vi "UsuarioContrasena.vi"() -> ()   [LabVIEW 2020]
panel:
  in  "stop":bool
  in  "Table Control":string[][](table)
  in  "Contraseña":string
  in  "Nombre":string
  out "Confirmado":bool
  out "Nombre confirmado":string
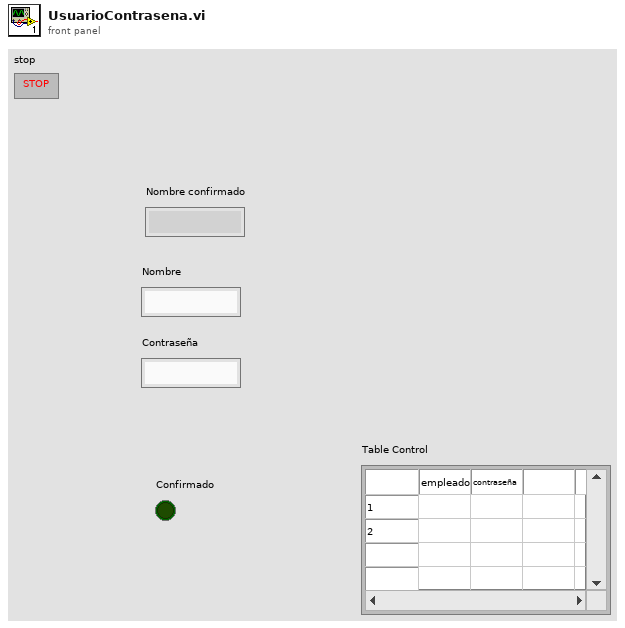
[diagram p1: front panel]
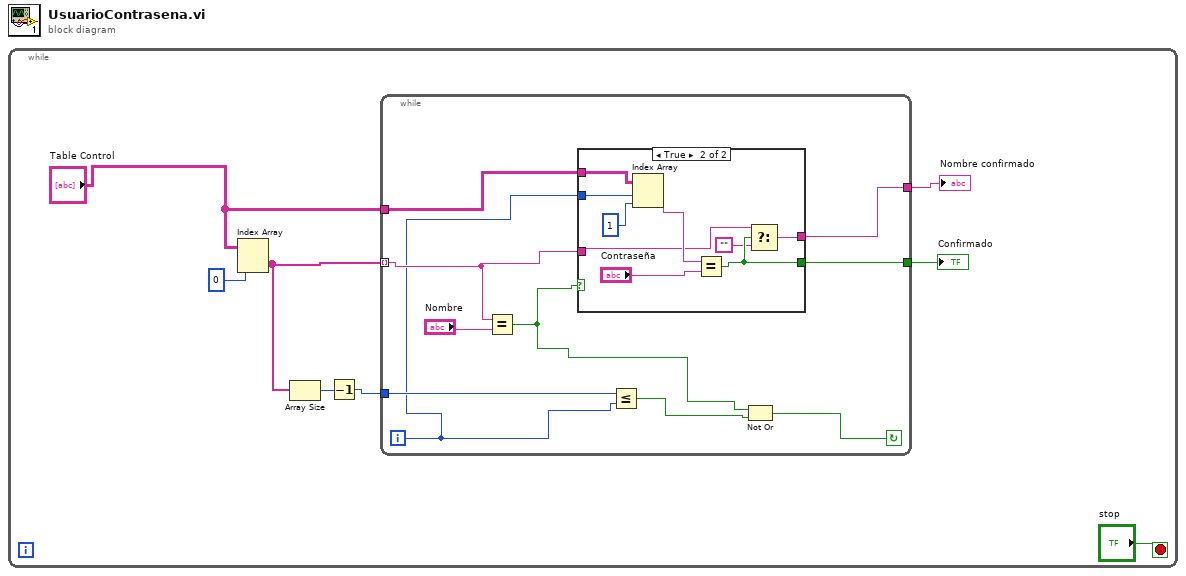
[diagram p0: block diagram]
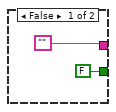
[diagram p2: hidden frame]
diagram:
  n1 = while {
    stop <- "stop" stop-if-true
    n2 = Index Array "Index Array"(array="Table Control", index (col)=0 ("disabled index (col)")) -> (element=w5:string[])  [unwired: 1 in]
    n3 = Array Size(array=w5) -> (size(s)=w3:i32)
    n4 = Decrement(x=w3) -> (x-1=w4:i32)
    n5 = while {
      tunnel: w4 -> [w16]
      tunnel: w5 -> [w14] mode=indexing
      tunnel: [w13] -> w6
      tunnel: [w12] -> w7
      tunnel: "Table Control" -> [w11]
      i -> [w10]
      stop <- w18 continue-if-true
      n6 = Equal?(x=w14, y="Nombre") -> (x = y?=w9:bool)
      n7 = case shown="True" w9 {
        tunnel: w11 -> [_ w23]
        tunnel: w14 -> [_ w26]
        tunnel: [FALSE w25] -> w13
        tunnel: ["" w24] -> w12
        tunnel: w10 -> [_ w22]
        frame False {
        }
        frame True {
          n8 = Index Array(array=w23, index (row)=w22, index (col)=1) -> (element=w27:string)
          n9 = Equal?(x=w27, y="Contraseña") -> (x = y?=w25:bool)
          n10 = Select(t=w26, s=w25, f="") -> (s? t:f=w24:string)
        }
      }
      n11 = Less Or Equal?(x=w16, y=w10) -> (x <= y?=w17:bool)
      n12 = Not Or(1:w17, 2:w9) -> (0:w18:bool)
    }
    "Confirmado" <- w6
    "Nombre confirmado" <- w7
  }
